vi "nanocal -- nuclear schottky fit V8.vi"() -> ()   [LabVIEW 2021] (continued)
  in  "filenames":u16(ring)=29 caption="files" items=["IDS0158_210310_RAW_cal_CeCoIn5_2nd_047_12T_fsweep_final_0.12K_0deg_Tdep_raw_.dat", "IDS0183_210310_RAW_cal_CeCoIn5_2nd_071_12T_0.120K_90deg_Tdep_raw_.dat", "IDS0311_210901_RAW_cal_CeCoIn5_4th_040(126)_C(f)_12T_0.120K_45deg_Tdep_raw_.dat", "IDS0359_210907_RAW_cal_CeCoIn5_4th_089_C(f)_12.0T_0.12K_60deg_Tdep_raw_.dat", "IDS0412_220525_RAW_cal_CeCoIn5_5th_017_0T_0deg__fSweep_0.12K_raw_.dat", "IDS0431_220527_RAW_cal_CeCoIn5_5th_036_10T_0deg__fSweep_0.12K_raw_.dat", "IDS0442_220528_RAW_cal_CeCoIn5_5th_047_6T_0deg__fSweep_0.12K_raw_.dat", "IDS0464_220530_RAW_cal_CeCoIn5_5th_069_4T_0deg__fSweep_0.12K_raw_.dat", "IDS0486_220602_RAW_cal_CeCoIn5_5th_091_10T_45deg__fSweep_0.12K_raw_.dat", "IDS0495_220602_RAW_cal_CeCoIn5_5th_099_8T_45deg__fSweep_0.12K_raw_.dat", "IDS0510_220603_RAW_cal_CeCoIn5_5th_114_6T_45deg__fSweep_0.12K_raw_.dat", "IDS0526_220605_RAW_cal_CeCoIn5_5th_130_4T_45deg__fSweep_0.12K_raw_.dat", "IDS0544_220606_RAW_cal_CeCoIn5_5th_148_2T_45deg__fSweep_0.12K_raw_.dat", "IDS0561_220607_RAW_cal_CeCoIn5_5th_165_2T_0deg_fSweep_0.12K_raw_.dat", "IDS0581_220608_RAW_cal_CeCoIn5_5th_185_2T_90deg_fSweep_0.12K_raw_.dat", "IDS0598_220609_RAW_cal_CeCoIn5_5th_202_4T_90deg_fSweep_0.12K_raw_.dat", "IDS0627_220611_RAW_cal_CeCoIn5_5th_231_10T_90deg_fSweep_0.12K_raw_.dat", "IDS0643_220612_RAW_cal_CeCoIn5_5th_247_6T_90deg_fSweep_0.12K_raw_.dat", "IDS0336_210904_RAW_cal_CeCoIn5_4th_065_C(f)_5.0T_0.122K_90deg_Tdep_raw_.dat", "IDS0346_210904_RAW_cal_CeCoIn5_4th_075_C(f)_8.0T_0.122K_90deg_Tdep_raw_.dat", "IDS0378_210909_RAW_cal_CeCoIn5_4th_108_C(f)_8.0T_0.122K_0deg_Tdep_raw_.dat", "IDS0300_210427_RAW_cal_CeCoIn5_4th_029(113)_C(f)_12T_0.14K_30deg_NEW_Tdep_raw_.dat", "IDS0184_210310_RAW_cal_CeCoIn5_2nd_072_12T_0.148K_90deg_Tdep_raw_.dat", "IDS0210_210310_RAW_cal_CeCoIn5_2nd_098_fsweep_6T_0.148K_Bdep_raw_.dat", "IDS0379_210909_RAW_cal_CeCoIn5_4th_109_C(f)_8.0T_0.148K_0deg_Tdep_raw_.dat", "IDS0159_210310_RAW_cal_CeCoIn5_2nd_048_12T_fsweep_0.15K_0deg_Tdep_raw_.dat", "IDS0360_210907_RAW_cal_CeCoIn5_4th_090_C(f)_12.0T_0.15K_60deg_Tdep_raw_.dat", "IDS0411_220525_RAW_cal_CeCoIn5_5th_016_0T_0deg__fSweep_0.15K_raw_.dat", "IDS0427_220526_RAW_cal_CeCoIn5_5th_032_10T_0deg__fSweep_0.15K_raw_.dat", "IDS0443_220528_RAW_cal_CeCoIn5_5th_048_6T_0deg__fSweep_0.15K_raw_.dat", "IDS0463_220530_RAW_cal_CeCoIn5_5th_068_4T_0deg__fSweep_0.15K_raw_.dat", "IDS0487_220602_RAW_cal_CeCoIn5_5th_092_10T_45deg__fSweep_0.15K_raw_.dat", "IDS0496_220602_RAW_cal_CeCoIn5_5th_100_8T_45deg__fSweep_0.15K_raw_.dat", "IDS0509_220603_RAW_cal_CeCoIn5_5th_113_6T_45deg__fSweep_0.15K_raw_.dat", "IDS0525_220605_RAW_cal_CeCoIn5_5th_129_4T_45deg__fSweep_0.15K_raw_.dat", "IDS0543_220606_RAW_cal_CeCoIn5_5th_147_2T_45deg__fSweep_0.15K_raw_.dat", "IDS0560_220607_RAW_cal_CeCoIn5_5th_164_2T_0deg_fSweep_0.15K_raw_.dat", "IDS0580_220608_RAW_cal_CeCoIn5_5th_184_2T_90deg_fSweep_0.15K_raw_.dat", "IDS0597_220608_RAW_cal_CeCoIn5_5th_201_4T_90deg_fSweep_0.15K_raw_.dat", "IDS0626_220611_RAW_cal_CeCoIn5_5th_230_10T_90deg_fSweep_0.15K_raw_.dat", "IDS0642_220612_RAW_cal_CeCoIn5_5th_246_6T_90deg_fSweep_0.15K_raw_.dat", "IDS0310_210901_RAW_cal_CeCoIn5_4th_039(125)_C(f)_12T_0.157K_45deg_Tdep_raw_.dat", "IDS0337_210904_RAW_cal_CeCoIn5_4th_066_C(f)_5.0T_0.157K_90deg_Tdep_raw_.dat", "IDS0347_210906_RAW_cal_CeCoIn5_4th_076_C(f)_8.0T_0.157K_90deg_Tdep_raw_.dat", "IDS0305_210831_RAW_cal_CeCoIn5_4th_034(110)_C(f)_12T_0.16K_30deg_NEW_Tdep_raw_.dat", "IDS0361_210908_RAW_cal_CeCoIn5_4th_091_C(f)_12.0T_0.168K_60deg_Tdep_raw_.dat", "IDS0380_210909_RAW_cal_CeCoIn5_4th_110_C(f)_8.0T_0.168K_0deg_Tdep_raw_.dat", "IDS0304_210831_RAW_cal_CeCoIn5_4th_033(112)_C(f)_12T_0.17K_30deg_NEW_Tdep_raw_.dat", "IDS0312_210901_RAW_cal_CeCoIn5_4th_041(127)_C(f)_12T_0.170K_45deg_Tdep_raw_.dat", "IDS0338_210904_RAW_cal_CeCoIn5_4th_067_C(f)_5.0T_0.170K_90deg_Tdep_raw_.dat", "IDS0410_220525_RAW_cal_CeCoIn5_5th_015_0T_0deg__fSweep_0.17K_raw_.dat", "IDS0432_220527_RAW_cal_CeCoIn5_5th_037_10T_0deg__fSweep_0.17K_raw_.dat", "IDS0444_220528_RAW_cal_CeCoIn5_5th_049_6T_0deg__fSweep_0.17K_raw_.dat", "IDS0462_220530_RAW_cal_CeCoIn5_5th_067_4T_0deg__fSweep_0.17K_raw_.dat", "IDS0485_220601_RAW_cal_CeCoIn5_5th_090_10T_45deg__fSweep_0.17K_raw_.dat", "IDS0497_220603_RAW_cal_CeCoIn5_5th_101_8T_45deg__fSweep_0.17K_raw_.dat", "IDS0511_220604_RAW_cal_CeCoIn5_5th_115_6T_45deg__fSweep_0.17K_raw_.dat", "IDS0524_220605_RAW_cal_CeCoIn5_5th_128_4T_45deg__fSweep_0.17K_raw_.dat", "IDS0542_220606_RAW_cal_CeCoIn5_5th_146_2T_45deg__fSweep_0.17K_raw_.dat", "IDS0559_220607_RAW_cal_CeCoIn5_5th_163_2T_0deg_fSweep_0.17K_raw_.dat", "IDS0579_220608_RAW_cal_CeCoIn5_5th_183_2T_90deg_fSweep_0.17K_raw_.dat", "IDS0596_220608_RAW_cal_CeCoIn5_5th_200_4T_90deg_fSweep_0.17K_raw_.dat", "IDS0625_220611_RAW_cal_CeCoIn5_5th_229_10T_90deg_fSweep_0.17K_raw_.dat", "IDS0641_220612_RAW_cal_CeCoIn5_5th_245_6T_90deg_fSweep_0.17K_raw_.dat", "IDS0348_210906_RAW_cal_CeCoIn5_4th_077_C(f)_8.0T_0.178K_90deg_Tdep_raw_.dat", "IDS0181_210310_RAW_cal_CeCoIn5_2nd_070_12T_0.179K_90deg_fsweep_Tdep_raw_.dat", "IDS0160_210310_RAW_cal_CeCoIn5_2nd_049_12T_fsweep_0.18K_0deg_Tdep_raw_.dat", "IDS0424_220526_RAW_cal_CeCoIn5_5th_029_10T_0deg__fSweep_0.19K_raw_.dat", "IDS0185_210310_RAW_cal_CeCoIn5_2nd_073_12T_0.197K_90deg_Tdep_raw_.dat", "IDS0208_210310_RAW_cal_CeCoIn5_2nd_096_Hsweep_0.197K_Bdep_raw_.dat", "IDS0209_210310_RAW_cal_CeCoIn5_2nd_097_Hsweep_0.197K_Bdep_raw_.dat", "IDS0211_210310_RAW_cal_CeCoIn5_2nd_099_fsweep_9T_0.197K_Bdep_raw_.dat", "IDS0212_210310_RAW_cal_CeCoIn5_2nd_100_fsweep_11T_0.197K_Bdep_raw_.dat", "IDS0213_210310_RAW_cal_CeCoIn5_2nd_101_fsweep_10T_0.197K_Bdep_raw_.dat", "IDS0214_210310_RAW_cal_CeCoIn5_2nd_102_fsweep_8T_0.197K_Bdep_raw_.dat", "IDS0215_210310_RAW_cal_CeCoIn5_2nd_103_fsweep_7T_0.197K_Bdep_raw_.dat", "IDS0216_210310_RAW_cal_CeCoIn5_2nd_104_fsweep_5T_0.197K_Bdep_raw_.dat", "IDS0217_210310_RAW_cal_CeCoIn5_2nd_105_fsweep_0T_0.197K_Bdep_raw_.dat", "IDS0330_210901_RAW_cal_CeCoIn5_4th_059_C(f)_1T_0.197K_90deg_Bdep_raw_.dat", "IDS0331_210901_RAW_cal_CeCoIn5_4th_060_C(f)_2T_0.197K_90deg_Bdep_raw_.dat", "IDS0335_210904_RAW_cal_CeCoIn5_4th_064_C(f)_5.0T_0.197K_90deg_Tdep_raw_.dat", "IDS0362_210908_RAW_cal_CeCoIn5_4th_092_C(f)_12.0T_0.197K_60deg_Tdep_raw_.dat", "IDS0377_210909_RAW_cal_CeCoIn5_4th_107_C(f)_8.0T_0.197K_0deg_Tdep_raw_.dat", "IDS0161_210310_RAW_cal_CeCoIn5_2nd_050_12T_fsweep_0.20K_0deg_Tdep_raw_.dat", "IDS0303_210831_RAW_cal_CeCoIn5_4th_032(114)_C(f)_12T_0.20K_30deg_NEW_Tdep_raw_.dat", "IDS0313_210901_RAW_cal_CeCoIn5_4th_042(128)_C(f)_12T_0.200K_45deg_Tdep_raw_.dat", "IDS0349_210906_RAW_cal_CeCoIn5_4th_078_C(f)_8.0T_0.20K_90deg_Tdep_raw_.dat", "IDS0407_220525_RAW_cal_CeCoIn5_5th_012_0T_0deg__fSweep_0.20K_raw_.dat", "IDS0441_220527_RAW_cal_CeCoIn5_5th_045_6T_0deg__fSweep_0.20K_raw_.dat", "IDS0458_220529_RAW_cal_CeCoIn5_5th_063_4T_0deg__fSweep_0.20K_raw_.dat", "IDS0477_220601_RAW_cal_CeCoIn5_5th_082_10T_45deg__fSweep_0.20K_raw_.dat", "IDS0493_220602_RAW_cal_CeCoIn5_5th_097_8T_45deg__fSweep_0.20K_raw_.dat", "IDS0508_220603_RAW_cal_CeCoIn5_5th_112_6T_45deg__fSweep_0.20K_raw_.dat", "IDS0523_220604_RAW_cal_CeCoIn5_5th_127_4T_45deg__fSweep_0.20K_raw_.dat", "IDS0540_220605_RAW_cal_CeCoIn5_5th_144_2T_45deg__fSweep_0.20K_raw_.dat", "IDS0562_220607_RAW_cal_CeCoIn5_5th_166_2T_0deg_fSweep_0.20K_raw_.dat", "IDS0578_220608_RAW_cal_CeCoIn5_5th_182_2T_90deg_fSweep_0.20K_raw_.dat", "IDS0595_220608_RAW_cal_CeCoIn5_5th_199_4T_90deg_fSweep_0.20K_raw_.dat", "IDS0624_220611_RAW_cal_CeCoIn5_5th_228_10T_90deg_fSweep_0.20K_raw_.dat", "IDS0640_220612_RAW_cal_CeCoIn5_5th_244_6T_90deg_fSweep_0.20K_raw_.dat", "IDS0186_210310_RAW_cal_CeCoIn5_2nd_074_12T_0.249K_90deg_Tdep_raw_.dat", "IDS0162_210310_RAW_cal_CeCoIn5_2nd_051_12T_fsweep_0.25K_0deg_Tdep_raw_.dat", "IDS0302_210831_RAW_cal_CeCoIn5_4th_031(115)_C(f)_12T_0.25K_30deg_NEW_Tdep_raw_.dat", "IDS0363_210908_RAW_cal_CeCoIn5_4th_093_C(f)_12.0T_0.25K_60deg_Tdep_raw_.dat", "IDS0381_210909_RAW_cal_CeCoIn5_4th_111_C(f)_8.0T_0.25K_0deg_Tdep_raw_.dat", "IDS0408_220525_RAW_cal_CeCoIn5_5th_013_0T_0deg__fSweep_0.25K_raw_.dat", "IDS0425_220526_RAW_cal_CeCoIn5_5th_030_10T_0deg__fSweep_0.25K_raw_.dat", "IDS0445_220528_RAW_cal_CeCoIn5_5th_050_6T_0deg__fSweep_0.25K_raw_.dat", "IDS0459_220529_RAW_cal_CeCoIn5_5th_064_4T_0deg__fSweep_0.25K_raw_.dat", "IDS0478_220601_RAW_cal_CeCoIn5_5th_083_10T_45deg__fSweep_0.25K_raw_.dat", "IDS0494_220602_RAW_cal_CeCoIn5_5th_098_8T_45deg__fSweep_0.25K_raw_.dat", "IDS0512_220604_RAW_cal_CeCoIn5_5th_116_6T_45deg__fSweep_0.25K_raw_.dat", "IDS0527_220605_RAW_cal_CeCoIn5_5th_131_4T_45deg__fSweep_0.25K_raw_.dat", "IDS0541_220605_RAW_cal_CeCoIn5_5th_145_2T_45deg__fSweep_0.25K_raw_.dat", "IDS0563_220607_RAW_cal_CeCoIn5_5th_167_2T_0deg_fSweep_0.25K_raw_.dat", "IDS0582_220608_RAW_cal_CeCoIn5_5th_186_2T_90deg_fSweep_0.25K_raw_.dat", "IDS0599_220609_RAW_cal_CeCoIn5_5th_203_4T_90deg_fSweep_0.25K_raw_.dat", "IDS0628_220611_RAW_cal_CeCoIn5_5th_232_10T_90deg_fSweep_0.25K_raw_.dat", "IDS0644_220612_RAW_cal_CeCoIn5_5th_248_6T_90deg_fSweep_0.25K_raw_.dat", "IDS0314_210901_RAW_cal_CeCoIn5_4th_043(129)_C(f)_12T_0.255K_45deg_Tdep_raw_.dat", "IDS0339_210904_RAW_cal_CeCoIn5_4th_068_C(f)_5.0T_0.255K_90deg_Tdep_raw_.dat", "IDS0350_210906_RAW_cal_CeCoIn5_4th_079_C(f)_8.0T_0.26K_90deg_Tdep_raw_.dat", "IDS0163_210310_RAW_cal_CeCoIn5_2nd_052_12T_fsweep_0.30K_0deg_Tdep_raw_.dat", "IDS0187_210310_RAW_cal_CeCoIn5_2nd_075_12T_0.300K_90deg_Tdep_raw_.dat", "IDS0301_210831_RAW_cal_CeCoIn5_4th_030(116)_C(f)_12T_0.30K_30deg_NEW_Tdep_raw_.dat", "IDS0315_210901_RAW_cal_CeCoIn5_4th_044(130)_C(f)_12T_0.300K_45deg_Tdep_raw_.dat", "IDS0382_210909_RAW_cal_CeCoIn5_4th_112_C(f)_8.0T_0.30K_0deg_Tdep_raw_.dat", "IDS0409_220525_RAW_cal_CeCoIn5_5th_014_0T_0deg__fSweep_0.30K_raw_.dat", "IDS0426_220526_RAW_cal_CeCoIn5_5th_031_10T_0deg__fSweep_0.30K_raw_.dat", "IDS0446_220528_RAW_cal_CeCoIn5_5th_051_6T_0deg__fSweep_0.30K_raw_.dat", "IDS0460_220529_RAW_cal_CeCoIn5_5th_065_4T_0deg__fSweep_0.30K_raw_.dat", "IDS0479_220601_RAW_cal_CeCoIn5_5th_084_10T_45deg__fSweep_0.30K_raw_.dat", "IDS0498_220603_RAW_cal_CeCoIn5_5th_102_8T_45deg__fSweep_0.30K_raw_.dat", "IDS0513_220604_RAW_cal_CeCoIn5_5th_117_6T_45deg__fSweep_0.30K_raw_.dat", "IDS0528_220605_RAW_cal_CeCoIn5_5th_132_4T_45deg__fSweep_0.30K_raw_.dat", "IDS0545_220606_RAW_cal_CeCoIn5_5th_149_2T_45deg__fSweep_0.30K_raw_.dat", "IDS0564_220607_RAW_cal_CeCoIn5_5th_168_2T_0deg_fSweep_0.30K_raw_.dat", "IDS0583_220608_RAW_cal_CeCoIn5_5th_187_2T_90deg_fSweep_0.30K_raw_.dat", "IDS0629_220611_RAW_cal_CeCoIn5_5th_233_10T_90deg_fSweep_0.30K_raw_.dat", "IDS0645_220612_RAW_cal_CeCoIn5_5th_249_6T_90deg_fSweep_0.30K_raw_.dat", "IDS0656_220614_RAW_cal_CeCoIn5_5th_260_4T_90deg_fSweep_0.30K_raw_.dat", "IDS0364_210908_RAW_cal_CeCoIn5_4th_094_C(f)_12.0T_0.307K_60deg_Tdep_raw_.dat", "IDS0340_210904_RAW_cal_CeCoIn5_4th_069_C(f)_5.0T_0.308K_90deg_Tdep_raw_.dat", "IDS0351_210906_RAW_cal_CeCoIn5_4th_080_C(f)_8.0T_0.31K_90deg_Tdep_raw_.dat", "IDS0164_210310_RAW_cal_CeCoIn5_2nd_053_12T_fsweep_0.36K_0deg_Tdep_raw_.dat", "IDS0188_210310_RAW_cal_CeCoIn5_2nd_076_12T_0.360K_90deg_Tdep_raw_.dat", "IDS0299_210427_RAW_cal_CeCoIn5_4th_028(117)_C(f)_12T_0.36K_30deg_NEW_Tdep_raw_.dat", "IDS0316_210901_RAW_cal_CeCoIn5_4th_045(131)_C(f)_12T_0.360K_45deg_Tdep_raw_.dat", "IDS0341_210904_RAW_cal_CeCoIn5_4th_070_C(f)_5.0T_0.360K_90deg_Tdep_raw_.dat", "IDS0352_210906_RAW_cal_CeCoIn5_4th_081_C(f)_8.0T_0.36K_90deg_Tdep_raw_.dat", "IDS0365_210908_RAW_cal_CeCoIn5_4th_095_C(f)_12.0T_0.36K_60deg_Tdep_raw_.dat", "IDS0383_210910_RAW_cal_CeCoIn5_4th_113_C(f)_8.0T_0.36K_0deg_Tdep_raw_.dat", "IDS0413_220525_RAW_cal_CeCoIn5_5th_018_0T_0deg__fSweep_0.36K_raw_.dat", "IDS0428_220526_RAW_cal_CeCoIn5_5th_033_10T_0deg__fSweep_0.36K_raw_.dat", "IDS0447_220528_RAW_cal_CeCoIn5_5th_052_6T_0deg__fSweep_0.36K_raw_.dat", "IDS0461_220529_RAW_cal_CeCoIn5_5th_066_4T_0deg__fSweep_0.36K_raw_.dat", "IDS0480_220601_RAW_cal_CeCoIn5_5th_085_10T_45deg__fSweep_0.36K_raw_.dat", "IDS0499_220603_RAW_cal_CeCoIn5_5th_103_8T_45deg__fSweep_0.36K_raw_.dat", "IDS0514_220604_RAW_cal_CeCoIn5_5th_118_6T_45deg__fSweep_0.36K_raw_.dat", "IDS0529_220605_RAW_cal_CeCoIn5_5th_133_4T_45deg__fSweep_0.36K_raw_.dat", "IDS0546_220606_RAW_cal_CeCoIn5_5th_150_2T_45deg__fSweep_0.36K_raw_.dat", "IDS0565_220607_RAW_cal_CeCoIn5_5th_169_2T_0deg_fSweep_0.36K_raw_.dat", "IDS0584_220608_RAW_cal_CeCoIn5_5th_188_2T_90deg_fSweep_0.36K_raw_.dat", "IDS0601_220609_RAW_cal_CeCoIn5_5th_205_4T_90deg_fSweep_0.36K_raw_.dat", "IDS0630_220611_RAW_cal_CeCoIn5_5th_234_10T_90deg_fSweep_0.36K_raw_.dat", "IDS0646_220612_RAW_cal_CeCoIn5_5th_250_6T_90deg_fSweep_0.36K_raw_.dat", "IDS0429_220526_RAW_cal_CeCoIn5_5th_034_10T_0deg__fSweep_0.42K_raw_.dat", "IDS0448_220528_RAW_cal_CeCoIn5_5th_053_6T_0deg__fSweep_0.42K_raw_.dat", "IDS0481_220601_RAW_cal_CeCoIn5_5th_086_10T_45deg__fSweep_0.42K_raw_.dat", "IDS0500_220603_RAW_cal_CeCoIn5_5th_104_8T_45deg__fSweep_0.42K_raw_.dat", "IDS0530_220605_RAW_cal_CeCoIn5_5th_134_4T_45deg__fSweep_0.42K_raw_.dat", "IDS0547_220606_RAW_cal_CeCoIn5_5th_151_2T_45deg__fSweep_0.42K_raw_.dat", "IDS0566_220607_RAW_cal_CeCoIn5_5th_170_2T_0deg_fSweep_0.42K_raw_.dat", "IDS0585_220608_RAW_cal_CeCoIn5_5th_189_2T_90deg_fSweep_0.42K_raw_.dat", "IDS0602_220609_RAW_cal_CeCoIn5_5th_206_4T_90deg_fSweep_0.42K_raw_.dat", "IDS0631_220611_RAW_cal_CeCoIn5_5th_235_10T_90deg_fSweep_0.42K_raw_.dat", "IDS0647_220612_RAW_cal_CeCoIn5_5th_251_6T_90deg_fSweep_0.42K_raw_.dat", "IDS0165_210310_RAW_cal_CeCoIn5_2nd_054_12T_fsweep_0.43K_0deg_Tdep_raw_.dat", "IDS0189_210310_RAW_cal_CeCoIn5_2nd_077_12T_0.430K_90deg_Tdep_raw_.dat", "IDS0298_210427_RAW_cal_CeCoIn5_4th_027(118)_C(f)_12T_0.43K_30deg_NEW_Tdep_raw_.dat", "IDS0317_210901_RAW_cal_CeCoIn5_4th_046(132)_C(f)_12T_0.43K_45deg_Tdep_raw_.dat", "IDS0366_210908_RAW_cal_CeCoIn5_4th_096_C(f)_12.0T_0.43K_60deg_Tdep_raw_.dat", "IDS0384_210910_RAW_cal_CeCoIn5_4th_114_C(f)_8.0T_0.43K_0deg_Tdep_raw_.dat", "IDS0414_220525_RAW_cal_CeCoIn5_5th_019_0T_0deg__fSweep_0.43K_raw_.dat", "IDS0465_220530_RAW_cal_CeCoIn5_5th_070_4T_0deg__fSweep_0.43K_raw_.dat", "IDS0515_220604_RAW_cal_CeCoIn5_5th_119_6T_45deg__fSweep_0.43K_raw_.dat", "IDS0342_210904_RAW_cal_CeCoIn5_4th_071_C(f)_5.0T_0.438K_90deg_Tdep_raw_.dat", "IDS0353_210906_RAW_cal_CeCoIn5_4th_082_C(f)_8.0T_0.438K_90deg_Tdep_raw_.dat", "IDS0190_210310_RAW_cal_CeCoIn5_2nd_078_12T_0.512K_90deg_Tdep_raw_.dat", "IDS0166_210310_RAW_cal_CeCoIn5_2nd_055_12T_fsweep_0.52K_0deg_Tdep_raw_.dat", "IDS0430_220526_RAW_cal_CeCoIn5_5th_035_10T_0deg__fSweep_0.52K_raw_.dat", "IDS0449_220528_RAW_cal_CeCoIn5_5th_054_6T_0deg__fSweep_0.52K_raw_.dat", "IDS0482_220601_RAW_cal_CeCoIn5_5th_087_10T_45deg__fSweep_0.52K_raw_.dat", "IDS0501_220603_RAW_cal_CeCoIn5_5th_105_8T_45deg__fSweep_0.52K_raw_.dat", "IDS0516_220604_RAW_cal_CeCoIn5_5th_120_6T_45deg__fSweep_0.52K_raw_.dat", "IDS0531_220605_RAW_cal_CeCoIn5_5th_135_4T_45deg__fSweep_0.52K_raw_.dat", "IDS0548_220606_RAW_cal_CeCoIn5_5th_152_2T_45deg__fSweep_0.52K_raw_.dat", "IDS0567_220607_RAW_cal_CeCoIn5_5th_171_2T_0deg_fSweep_0.52K_raw_.dat", "IDS0586_220608_RAW_cal_CeCoIn5_5th_190_2T_90deg_fSweep_0.52K_raw_.dat", "IDS0603_220609_RAW_cal_CeCoIn5_5th_207_4T_90deg_fSweep_0.52K_raw_.dat", "IDS0632_220611_RAW_cal_CeCoIn5_5th_236_10T_90deg_fSweep_0.52K_raw_.dat", "IDS0648_220613_RAW_cal_CeCoIn5_5th_252_6T_90deg_fSweep_0.52K_raw_.dat", "IDS0297_210427_RAW_cal_CeCoIn5_4th_026(119)_C(f)_12T_0.53K_30deg_NEW_Tdep_raw_.dat", "IDS0318_210901_RAW_cal_CeCoIn5_4th_047(133)_C(f)_12T_0.53K_45deg_Tdep_raw_.dat", "IDS0343_210904_RAW_cal_CeCoIn5_4th_072_C(f)_5.0T_0.53K_90deg_Tdep_raw_.dat", "IDS0354_210906_RAW_cal_CeCoIn5_4th_083_C(f)_8.0T_0.53K_90deg_Tdep_raw_.dat", "IDS0367_210908_RAW_cal_CeCoIn5_4th_097_C(f)_12.0T_0.53K_60deg_Tdep_raw_.dat", "IDS0385_210910_RAW_cal_CeCoIn5_4th_115_C(f)_8.0T_0.53K_0deg_Tdep_raw_.dat", "IDS0415_220525_RAW_cal_CeCoIn5_5th_020_0T_0deg__fSweep_0.53K_raw_.dat", "IDS0466_220530_RAW_cal_CeCoIn5_5th_071_4T_0deg__fSweep_0.53K_raw_.dat", "IDS0191_210310_RAW_cal_CeCoIn5_2nd_079_12T_0.610K_90deg_Tdep_raw_.dat", "IDS0167_210310_RAW_cal_CeCoIn5_2nd_056_12T_fsweep_0.62K_0deg_Tdep_raw_.dat", "IDS0296_210427_RAW_cal_CeCoIn5_4th_025(120)_C(f)_12T_0.62K_30deg_NEW_Tdep_raw_.dat", "IDS0319_210901_RAW_cal_CeCoIn5_4th_048(134)_C(f)_12T_0.62K_45deg_Tdep_raw_.dat", "IDS0344_210904_RAW_cal_CeCoIn5_4th_073_C(f)_5.0T_0.62K_90deg_Tdep_raw_.dat", "IDS0433_220527_RAW_cal_CeCoIn5_5th_038_10T_0deg__fSweep_0.62K_raw_.dat", "IDS0450_220528_RAW_cal_CeCoIn5_5th_055_6T_0deg__fSweep_0.62K_raw_.dat", "IDS0467_220530_RAW_cal_CeCoIn5_5th_072_4T_0deg__fSweep_0.62K_raw_.dat", "IDS0483_220601_RAW_cal_CeCoIn5_5th_088_10T_45deg__fSweep_0.62K_raw_.dat", "IDS0502_220603_RAW_cal_CeCoIn5_5th_106_8T_45deg__fSweep_0.62K_raw_.dat", "IDS0517_220604_RAW_cal_CeCoIn5_5th_121_6T_45deg__fSweep_0.62K_raw_.dat", "IDS0532_220605_RAW_cal_CeCoIn5_5th_136_4T_45deg__fSweep_0.62K_raw_.dat", "IDS0549_220606_RAW_cal_CeCoIn5_5th_153_2T_45deg__fSweep_0.62K_raw_.dat", "IDS0568_220607_RAW_cal_CeCoIn5_5th_172_2T_0deg_fSweep_0.62K_raw_.dat", "IDS0587_220608_RAW_cal_CeCoIn5_5th_191_2T_90deg_fSweep_0.62K_raw_.dat", "IDS0604_220609_RAW_cal_CeCoIn5_5th_208_4T_90deg_fSweep_0.62K_raw_.dat", "IDS0618_220610_RAW_cal_CeCoIn5_5th_222_8T_90deg_fSweep_0.62K_raw_.dat", "IDS0633_220611_RAW_cal_CeCoIn5_5th_237_10T_90deg_fSweep_0.62K_raw_.dat", "IDS0649_220613_RAW_cal_CeCoIn5_5th_253_6T_90deg_fSweep_0.62K_raw_.dat", "IDS0368_210908_RAW_cal_CeCoIn5_4th_098_C(f)_12.0T_0.63K_60deg_Tdep_raw_.dat", "IDS0386_210910_RAW_cal_CeCoIn5_4th_116_C(f)_8.0T_0.63K_0deg_Tdep_raw_.dat", "IDS0416_220525_RAW_cal_CeCoIn5_5th_021_0T_0deg__fSweep_0.63K_raw_.dat", "IDS0220_210310_RAW_cal_CeCoIn5_2nd_108_fsweep_0T_0.677K_Bdep_raw_.dat", "IDS0168_210310_RAW_cal_CeCoIn5_2nd_057_12T_fsweep_0.81K_0deg_Tdep_raw_.dat", "IDS0192_210310_RAW_cal_CeCoIn5_2nd_080_12T_0.810K_90deg_Tdep_raw_.dat", "IDS0434_220527_RAW_cal_CeCoIn5_5th_039_10T_0deg__fSweep_0.82K_raw_.dat", "IDS0451_220528_RAW_cal_CeCoIn5_5th_056_6T_0deg__fSweep_0.82K_raw_.dat", "IDS0468_220530_RAW_cal_CeCoIn5_5th_073_4T_0deg__fSweep_0.82K_raw_.dat", "IDS0484_220601_RAW_cal_CeCoIn5_5th_089_10T_45deg__fSweep_0.82K_raw_.dat", "IDS0503_220603_RAW_cal_CeCoIn5_5th_107_8T_45deg__fSweep_0.82K_raw_.dat", "IDS0518_220604_RAW_cal_CeCoIn5_5th_122_6T_45deg__fSweep_0.82K_raw_.dat", "IDS0533_220605_RAW_cal_CeCoIn5_5th_137_4T_45deg__fSweep_0.82K_raw_.dat", "IDS0550_220606_RAW_cal_CeCoIn5_5th_154_2T_45deg__fSweep_0.82K_raw_.dat", "IDS0569_220607_RAW_cal_CeCoIn5_5th_173_2T_0deg_fSweep_0.82K_raw_.dat", "IDS0588_220608_RAW_cal_CeCoIn5_5th_192_2T_90deg_fSweep_0.82K_raw_.dat", "IDS0605_220609_RAW_cal_CeCoIn5_5th_209_4T_90deg_fSweep_0.82K_raw_.dat", "IDS0612_220610_RAW_cal_CeCoIn5_5th_216_5T_90deg_fSweep_0.82K_raw_.dat", "IDS0634_220612_RAW_cal_CeCoIn5_5th_238_10T_90deg_fSweep_0.82K_raw_.dat", "IDS0650_220613_RAW_cal_CeCoIn5_5th_254_6T_90deg_fSweep_0.82K_raw_.dat", "IDS0295_210427_RAW_cal_CeCoIn5_4th_024(121)_C(f)_12T_0.83K_30deg_NEW_Tdep_raw_.dat", "IDS0320_210901_RAW_cal_CeCoIn5_4th_049(135)_C(f)_12T_0.83K_45deg_Tdep_raw_.dat", "IDS0355_210906_RAW_cal_CeCoIn5_4th_085_C(f)_8.0T_0.83K_90deg_Tdep_raw_.dat", "IDS0369_210908_RAW_cal_CeCoIn5_4th_099_C(f)_12.0T_0.83K_60deg_Tdep_raw_.dat", "IDS0387_210910_RAW_cal_CeCoIn5_4th_117_C(f)_8.0T_0.83K_0deg_Tdep_raw_.dat", "IDS0417_220525_RAW_cal_CeCoIn5_5th_022_0T_0deg__fSweep_0.83K_raw_.dat", "IDS0219_210310_RAW_cal_CeCoIn5_2nd_107_fsweep_0T_1.0K_Bdep_raw_.dat", "IDS0193_210310_RAW_cal_CeCoIn5_2nd_081_12T_1.1K_90deg_Tdep_raw_.dat", "IDS0606_220609_RAW_cal_CeCoIn5_5th_210_4T_90deg_fSweep_1.10K_raw_.dat", "IDS0169_210310_RAW_cal_CeCoIn5_2nd_058_12T_fsweep_1.12K_0deg_Tdep_raw_.dat", "IDS0418_220525_RAW_cal_CeCoIn5_5th_023_0T_0deg__fSweep_1.12K_raw_.dat", "IDS0435_220527_RAW_cal_CeCoIn5_5th_040_10T_0deg__fSweep_1.12K_raw_.dat", "IDS0452_220528_RAW_cal_CeCoIn5_5th_057_6T_0deg__fSweep_1.12K_raw_.dat", "IDS0469_220530_RAW_cal_CeCoIn5_5th_074_4T_0deg__fSweep_1.12K_raw_.dat", "IDS0488_220602_RAW_cal_CeCoIn5_5th_093_10T_45deg__fSweep_1.12K_raw_.dat", "IDS0504_220603_RAW_cal_CeCoIn5_5th_108_8T_45deg__fSweep_1.12K_raw_.dat", "IDS0519_220604_RAW_cal_CeCoIn5_5th_123_6T_45deg__fSweep_1.12K_raw_.dat", "IDS0534_220605_RAW_cal_CeCoIn5_5th_138_4T_45deg__fSweep_1.12K_raw_.dat", "IDS0551_220606_RAW_cal_CeCoIn5_5th_155_2T_45deg__fSweep_1.12K_raw_.dat", "IDS0570_220607_RAW_cal_CeCoIn5_5th_174_2T_0deg_fSweep_1.12K_raw_.dat", "IDS0589_220608_RAW_cal_CeCoIn5_5th_193_2T_90deg_fSweep_1.12K_raw_.dat", "IDS0613_220610_RAW_cal_CeCoIn5_5th_217_5T_90deg_fSweep_1.12K_raw_.dat", "IDS0619_220610_RAW_cal_CeCoIn5_5th_223_8T_90deg_fSweep_1.12K_raw_.dat", "IDS0635_220612_RAW_cal_CeCoIn5_5th_239_10T_90deg_fSweep_1.12K_raw_.dat", "IDS0651_220613_RAW_cal_CeCoIn5_5th_255_6T_90deg_fSweep_1.12K_raw_.dat", "IDS0294_210427_RAW_cal_CeCoIn5_4th_023(122)_C(f)_12T_1.13K_30deg_NEW_Tdep_raw_.dat", "IDS0321_210901_RAW_cal_CeCoIn5_4th_050(136)_C(f)_12T_1.13K_45deg_Tdep_raw_.dat", "IDS0370_210908_RAW_cal_CeCoIn5_4th_100_C(f)_12.0T_1.13K_60deg_Tdep_raw_.dat", "IDS0388_210910_RAW_cal_CeCoIn5_4th_118_C(f)_8.0T_1.13K_0deg_Tdep_raw_.dat", "IDS0391_210910_RAW_cal_CeCoIn5_4th_121_C(f)_8.0T_1.25K_0deg_Tdep_raw_.dat", "IDS0439_220527_RAW_cal_CeCoIn5_5th_044_10T_0deg__fSweep_1.28K_raw_.dat", "IDS0395_210910_RAW_cal_CeCoIn5_4th_125_C(f)_8.0T_1.31K_0deg_Tdep_raw_.dat", "IDS0392_210910_RAW_cal_CeCoIn5_4th_122_C(f)_8.0T_1.39K_0deg_Tdep_raw_.dat", "IDS0556_220606_RAW_cal_CeCoIn5_5th_160_4T_45deg__fSweep_1.50K_raw_.dat", "IDS0389_210910_RAW_cal_CeCoIn5_4th_119_C(f)_8.0T_1.52K_0deg_Tdep_raw_.dat", "IDS0218_210310_RAW_cal_CeCoIn5_2nd_106_fsweep_0T_1.55K_Bdep_raw_.dat", "IDS0590_220608_RAW_cal_CeCoIn5_5th_194_2T_90deg_fSweep_1.60K_raw_.dat", "IDS0607_220609_RAW_cal_CeCoIn5_5th_211_4T_90deg_fSweep_1.60K_raw_.dat", "IDS0453_220529_RAW_cal_CeCoIn5_5th_058_6T_0deg__fSweep_1.70K_raw_.dat", "IDS0535_220605_RAW_cal_CeCoIn5_5th_139_4T_45deg__fSweep_1.70K_raw_.dat", "IDS0170_210310_RAW_cal_CeCoIn5_2nd_059_12T_fsweep_1.80K_0deg_Tdep_raw_.dat", "IDS0194_210310_RAW_cal_CeCoIn5_2nd_082_12T_1.8K_90deg_Tdep_raw_.dat", "IDS0293_210427_RAW_cal_CeCoIn5_4th_022(123)_C(f)_12T_1.90K_30deg_NEW_Tdep_raw_.dat", "IDS0322_210901_RAW_cal_CeCoIn5_4th_051(137)_C(f)_12T_1.90K_45deg_Tdep_raw_.dat", "IDS0371_210908_RAW_cal_CeCoIn5_4th_101_C(f)_12.0T_1.90K_60deg_Tdep_raw_.dat", "IDS0390_210910_RAW_cal_CeCoIn5_4th_120_C(f)_8.0T_1.90K_0deg_Tdep_raw_.dat", "IDS0419_220525_RAW_cal_CeCoIn5_5th_024_0T_0deg__fSweep_1.90K_raw_.dat", "IDS0436_220527_RAW_cal_CeCoIn5_5th_041_10T_0deg__fSweep_1.90K_raw_.dat", "IDS0454_220529_RAW_cal_CeCoIn5_5th_059_6T_0deg__fSweep_1.90K_raw_.dat", "IDS0470_220530_RAW_cal_CeCoIn5_5th_075_4T_0deg__fSweep_1.90K_raw_.dat", "IDS0489_220602_RAW_cal_CeCoIn5_5th_094_10T_45deg__fSweep_1.90K_raw_.dat", "IDS0505_220603_RAW_cal_CeCoIn5_5th_109_8T_45deg__fSweep_1.90K_raw_.dat", "IDS0520_220604_RAW_cal_CeCoIn5_5th_124_6T_45deg__fSweep_1.90K_raw_.dat", "IDS0536_220605_RAW_cal_CeCoIn5_5th_140_4T_45deg__fSweep_1.90K_raw_.dat", "IDS0552_220606_RAW_cal_CeCoIn5_5th_156_2T_45deg__fSweep_1.90K_raw_.dat", "IDS0571_220607_RAW_cal_CeCoIn5_5th_175_2T_0deg_fSweep_1.90K_raw_.dat", "IDS0608_220610_RAW_cal_CeCoIn5_5th_212_4T_90deg_fSweep_1.90K_raw_.dat", "IDS0614_220610_RAW_cal_CeCoIn5_5th_218_5T_90deg_fSweep_1.90K_raw_.dat", "IDS0620_220610_RAW_cal_CeCoIn5_5th_224_8T_90deg_fSweep_1.90K_raw_.dat", "IDS0636_220612_RAW_cal_CeCoIn5_5th_240_10T_90deg_fSweep_1.90K_raw_.dat", "IDS0652_220613_RAW_cal_CeCoIn5_5th_256_6T_90deg_fSweep_1.90K_raw_.dat", "IDS0420_220525_RAW_cal_CeCoIn5_5th_025_0T_0deg__fSweep_2.10K_raw_.dat", "IDS0421_220525_RAW_cal_CeCoIn5_5th_026_0T_0deg__fSweep_2.30K_raw_.dat", "IDS0471_220530_RAW_cal_CeCoIn5_5th_076_4T_0deg__fSweep_2.30K_raw_.dat", "IDS0553_220606_RAW_cal_CeCoIn5_5th_157_2T_45deg__fSweep_2.30K_raw_.dat", "IDS0572_220607_RAW_cal_CeCoIn5_5th_176_2T_0deg_fSweep_2.30K_raw_.dat", "IDS0591_220608_RAW_cal_CeCoIn5_5th_195_2T_90deg_fSweep_2.30K_raw_.dat", "IDS0195_210310_RAW_cal_CeCoIn5_2nd_083_12T_3.0K_90deg_Tdep_raw_.dat", "IDS0472_220530_RAW_cal_CeCoIn5_5th_077_4T_0deg__fSweep_3.07K_raw_.dat", "IDS0171_210310_RAW_cal_CeCoIn5_2nd_060_12T_fsweep_3.10K_0deg_Tdep_raw_.dat", "IDS0306_210831_RAW_cal_CeCoIn5_4th_035(124)_C(f)_12T_3.10K_30deg_NEW_Tdep_raw_.dat", "IDS0323_210901_RAW_cal_CeCoIn5_4th_052(138)_C(f)_12T_3.10K_45deg_Tdep_raw_.dat", "IDS0422_220525_RAW_cal_CeCoIn5_5th_027_0T_0deg__fSweep_3.10K_raw_.dat", "IDS0437_220527_RAW_cal_CeCoIn5_5th_042_10T_0deg__fSweep_3.10K_raw_.dat", "IDS0455_220529_RAW_cal_CeCoIn5_5th_060_6T_0deg__fSweep_3.10K_raw_.dat", "IDS0490_220602_RAW_cal_CeCoIn5_5th_095_10T_45deg__fSweep_3.10K_raw_.dat", "IDS0506_220603_RAW_cal_CeCoIn5_5th_110_8T_45deg__fSweep_3.10K_raw_.dat", "IDS0521_220604_RAW_cal_CeCoIn5_5th_125_6T_45deg__fSweep_3.10K_raw_.dat", "IDS0537_220605_RAW_cal_CeCoIn5_5th_141_4T_45deg__fSweep_3.10K_raw_.dat", "IDS0554_220606_RAW_cal_CeCoIn5_5th_158_2T_45deg__fSweep_3.10K_raw_.dat", "IDS0573_220607_RAW_cal_CeCoIn5_5th_177_2T_0deg_fSweep_3.10K_raw_.dat", "IDS0592_220608_RAW_cal_CeCoIn5_5th_196_2T_90deg_fSweep_3.10K_raw_.dat", "IDS0609_220610_RAW_cal_CeCoIn5_5th_213_4T_90deg_fSweep_3.10K_raw_.dat", "IDS0615_220610_RAW_cal_CeCoIn5_5th_219_5T_90deg_fSweep_3.10K_raw_.dat", "IDS0621_220610_RAW_cal_CeCoIn5_5th_225_8T_90deg_fSweep_3.10K_raw_.dat", "IDS0637_220612_RAW_cal_CeCoIn5_5th_241_10T_90deg_fSweep_3.10K_raw_.dat", "IDS0653_220613_RAW_cal_CeCoIn5_5th_257_6T_90deg_fSweep_3.10K_raw_.dat", "IDS0372_210908_RAW_cal_CeCoIn5_4th_102_C(f)_12.0T_3.11K_60deg_Tdep_raw_.dat", "IDS0393_210910_RAW_cal_CeCoIn5_4th_123_C(f)_8.0T_3.11K_0deg_Tdep_raw_.dat", "IDS0172_210310_RAW_cal_CeCoIn5_2nd_061_12T_fsweep_5.50K_0deg_Tdep_raw_.dat", "IDS0196_210310_RAW_cal_CeCoIn5_2nd_084_12T_5.7K_90deg_Tdep_raw_.dat", "IDS0324_210901_RAW_cal_CeCoIn5_4th_053(139)_C(f)_12T_5.70K_45deg_Tdep_raw_.dat", "IDS0438_220527_RAW_cal_CeCoIn5_5th_043_10T_0deg__fSweep_5.70K_raw_.dat", "IDS0456_220529_RAW_cal_CeCoIn5_5th_061_6T_0deg__fSweep_5.70K_raw_.dat", "IDS0473_220531_RAW_cal_CeCoIn5_5th_078_4T_0deg__fSweep_5.70K_raw_.dat", "IDS0491_220602_RAW_cal_CeCoIn5_5th_096_10T_45deg__fSweep_5.70K_raw_.dat", "IDS0538_220605_RAW_cal_CeCoIn5_5th_142_4T_45deg__fSweep_5.70K_raw_.dat", "IDS0555_220606_RAW_cal_CeCoIn5_5th_159_2T_45deg__fSweep_5.70K_raw_.dat", "IDS0574_220607_RAW_cal_CeCoIn5_5th_178_2T_0deg_fSweep_5.70K_raw_.dat", "IDS0593_220608_RAW_cal_CeCoIn5_5th_197_2T_90deg_fSweep_5.70K_raw_.dat", "IDS0610_220610_RAW_cal_CeCoIn5_5th_214_4T_90deg_fSweep_5.70K_raw_.dat", "IDS0616_220610_RAW_cal_CeCoIn5_5th_220_5T_90deg_fSweep_5.70K_raw_.dat", "IDS0622_220610_RAW_cal_CeCoIn5_5th_226_8T_90deg_fSweep_5.70K_raw_.dat", "IDS0638_220612_RAW_cal_CeCoIn5_5th_242_10T_90deg_fSweep_5.70K_raw_.dat", "IDS0654_220613_RAW_cal_CeCoIn5_5th_258_6T_90deg_fSweep_5.70K_raw_.dat", "IDS0373_210908_RAW_cal_CeCoIn5_4th_103_C(f)_12.0T_5.75K_60deg_Tdep_raw_.dat", "IDS0394_210910_RAW_cal_CeCoIn5_4th_124_C(f)_8.0T_5.75K_0deg_Tdep_raw_.dat"]
  in  "folder":path=path "/Users/arkadyshekhter/Library/CloudStorage/Dropbox/shared_AkashAndreas/paper-CeCoIn5-spectroheat/Original RAW data"
  in  "file pattern":string="IDS*RAW*_raw_.dat"
  in  "string IN → Math! :~":bool
  in  "Math→ string OUT! :s":bool
